vi "3.4.vi"() -> ()   [LabVIEW 2018]
panel:
  out "삭제된 부분":string[](array[string])
  out "부분이 삭제된 배열":string[](array[string])
  out "출력 배열 2":string[](array[string])
  out "출력 배열":string[](array[string])
  out "원소":string
  out "크기":i32
  in  "배열":string[](array[string])
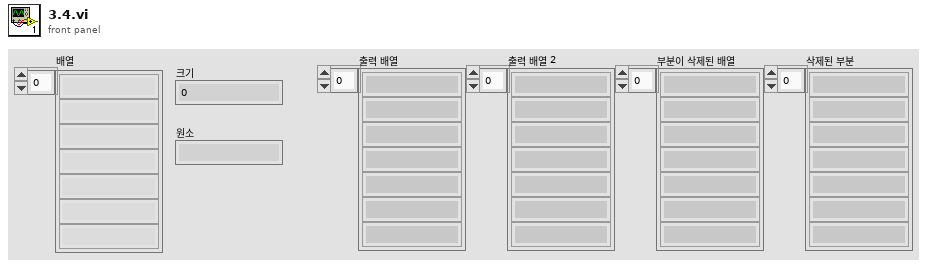
[diagram p1: front panel]
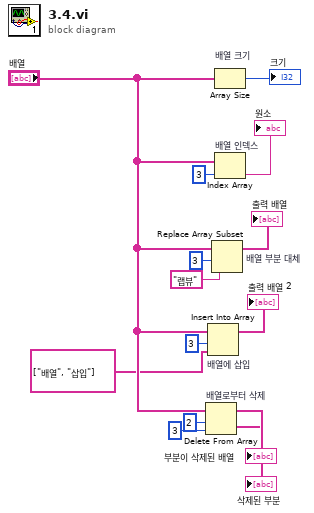
[diagram p0: block diagram]
diagram:
  n1 = Delete From Array "배열로부터 삭제"(array="배열", length=2 ("길이"), index=3 ("인덱스")) -> (deleted portion=→"삭제된 부분":string[], array with subset deleted=→"부분이 삭제된 배열":string[])
  n2 = Insert Into Array "배열에 삽입"(array="배열", index=3 ("인덱스"), new element=string[] ["배열", "삽입"]) -> (→"출력 배열 2":string[])
  n3 = Replace Array Subset "배열 부분 대체"(array="배열", new element="랩뷰" ("새 원소/부분배열"), index=3 ("인덱스")) -> (→"출력 배열":string[])
  n4 = Array Size "배열 크기"(array="배열") -> (size(s)=→"크기":i32)
  n5 = Index Array "배열 인덱스"(array="배열", index=3 ("인덱스")) -> (element=→"원소":string)
